vi "EN50160 Aggregation 10sec.vi"(0 "half-cycle frequency":T2, 4 "system info in":refnum<class "EP System Info.lvclass">, 5 "error in (no error)":errorcluster, 6 "reset? (F)":bool, 7 "voltage flags? (F)":bool[](array[boolean]), 8 "data timestamp":timestamp) -> (14 "10s values":T1, 18 "system info out":refnum<class "EP System Info.lvclass">, 19 "error out":errorcluster)   [LabVIEW 2014, in "NI_EP_Power Quality.lvlib"]
doc: "Calculates aggregated values of power quality parameters for specific intervals. You use the aggregated values for further evaluations according to EN 50160:2007. The aggregation methods are compliant with Class S in IEC 61000-4-30:2008. The aggregation is based on a 10-cycle time interval for a 50 Hz power system or 12-cycle time interval for a 60 Hz power system. There is no overlap between aggregation intervals. This VI automatically restarts accumulation at the beginning of the next 10/12-cycle time interval after the previous interval expires. You must manually select the polymorphic instance you want to use.\n\nThis VI supports measuring single-bus single-line or multiple-bus single-line systems."
uses:
  <vilib>/addons/Electrical Power/PQ/NI_EP_Power Quality.lvlib
  <vilib>/addons/Electrical Power/PQ/Common/Classes/System Info/EP System Info.lvclass
  <vilib>/addons/Electrical Power/PQ/Common/Controls/ep_Aggregation Settings.ctl
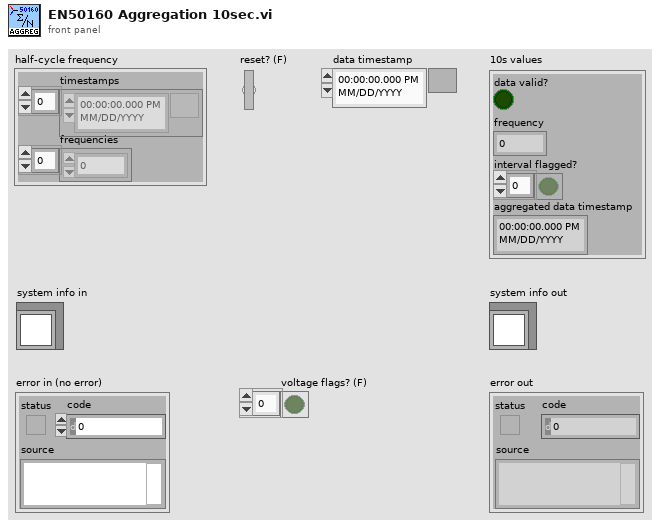
[diagram p1: front panel]
types:
  T1 = cluster{"data valid?":bool, "frequency":dbl, "interval flagged?":bool[], "aggregated data timestamp":timestamp}
  T2 = cluster{"timestamps":timestamp[], "frequencies":dbl[]}
  T3 = cluster{bool, "aggregated frequency":dbl, "aggregated voltage flags":bool[], "aggregated interval time stamp":timestamp}
  T4 = typedef "NI_EP_Power Quality.lvlib/ep_Aggregation Settings.ctl" = cluster{"interval":u32, "interval unit":enum16{"Runs", "Seconds", "Minutes", "Hours", "Days", "Weeks"}, "synchronization of intervals":enum16{"Not synchronized", "Interval rounded"}, "algorithm":enum16{"Average", "RMS"}}
  T5 = cluster{bool, "aggregated frequency":dbl, "aggregated voltage flags":bool[], "aggregated data time stamp":timestamp}
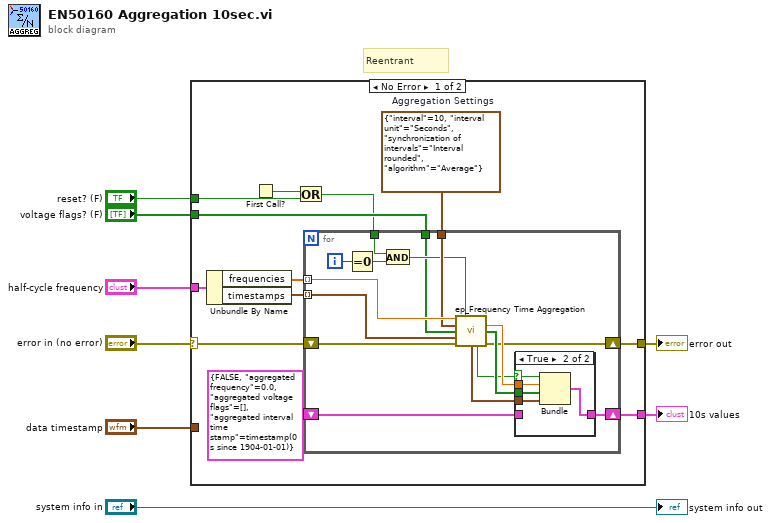
[diagram p0: block diagram]
diagram:
  # "Reentrant"
  n1 = case shown="No Error" "error in (no error)" {
    selector: "error in (no error)" -> [w19 w43]
    tunnel: [w13 _] -> w8
    tunnel: "reset? (F)" -> [w10 _]
    tunnel: [w15 w43] -> w6
    tunnel: "half-cycle frequency" -> [w18 _]
    tunnel: "data timestamp" -> [_ _]
    tunnel: "voltage flags? (F)" -> [w12 _]
    frame No Error {
      w20 = T4 {"interval"=10, "interval unit"=enum."Seconds", "synchronization of intervals"=enum."Interval rounded", "algorithm"=enum."Average"}  # Aggregation Settings
      n2 = Unbundle By Name(w18) -> ("frequencies"=w17:dbl[], "timestamps"=w16:timestamp[])
      n3 = First Call?() -> (First Call?: T/F=w11:bool)
      n4 = Or(x=w11, y=w10) -> (x .or. y?=w9:bool)
      n5 = for {
        tunnel: w9 -> [w32]
        tunnel: w20 -> [w31]
        shift-right: [w21] -> w15
        shift-left: w19 -> [w36]
        tunnel: w17 -> [w35] mode=indexing
        tunnel: w16 -> [w29] mode=indexing
        shift-right: [w27] -> w13
        shift-left: T3 {FALSE, "aggregated frequency"=0.0, "aggregated voltage flags"=[], "aggregated interval time stamp"=timestamp(0 s since 1904-01-01)} -> [w26]
        tunnel: w12 -> [w25]
        i -> [w34]
        n6 = Equal To 0?(x=w34) -> (x = 0?=w33:bool)
        n7 = And(x=w32, y=w33) -> (x .and. y?=w30:bool)
        n8 = call <vilib>:"ep_Frequency Time Aggregation.vi"("frequency (1/2) (half cycle)"=w35, "restart (F)"=w30, "aggregation settings"=w31, "voltage flags"=w25, "data time stamp"=w29, "error in (no error)"=w36) -> ("aggregated frequency"=w28:dbl, "aggregated voltage flags"=w24:bool[], "aggregated data time stamp"=w23:timestamp, "aggregated data valid?"=w22:bool, "error out"=w21:errorcluster)  [unwired: 5 in]
        n9 = case shown="True" w22 {
          selector: w22 -> [_ w42]
          tunnel: w28 -> [_ w41]
          tunnel: w23 -> [_ w39]
          tunnel: w24 -> [_ w40]
          tunnel: [w37 w38] -> w27
          tunnel: w26 -> [w37 _]
          frame False {
          }
          frame True {
            n10 = Bundle(w42, "aggregated frequency"=w41, "aggregated voltage flags"=w40, "aggregated data time stamp"=w39) -> (w38:T5)  [unwired: 1 in]
          }
        }
      }
    }
    frame Error {
    }
  }
  "error out" <- w6
  "10s values" <- w8
  "system info out" <- "system info in"
